vi "Test read mag.vi"() -> ()   [LabVIEW 2013]
uses:
  <vilib>/ni845x/ni845x.llb/ni845xControl.ctl
panel:
  out "whoami 2":u8 format="%.0x"
  out "whoami":u8 format="%.0x"
  out "dt":u32
  out "Waveform Chart":u8[](graph)
  in  "Stop":bool
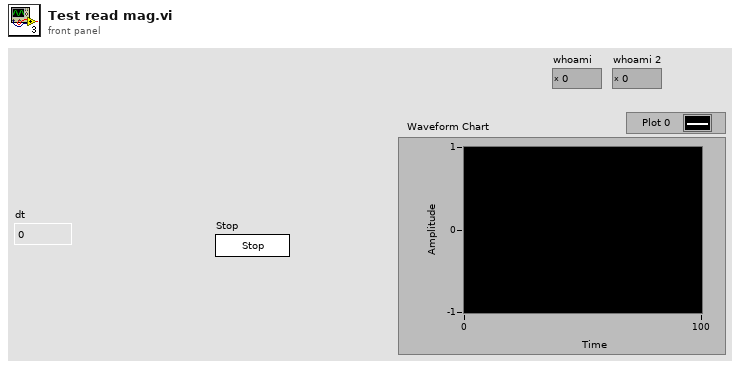
[diagram p1: front panel]
types:
  T1 = typedef "ni845xControl.ctl" = refnum<k21>
  T2 = typedef "AccelerometerSPI.ctl" = cluster{"Device":T1, "spi configuration":T3}
  T3 = typedef "ni845xSpiConfiguration.ctl" = refnum<k20>
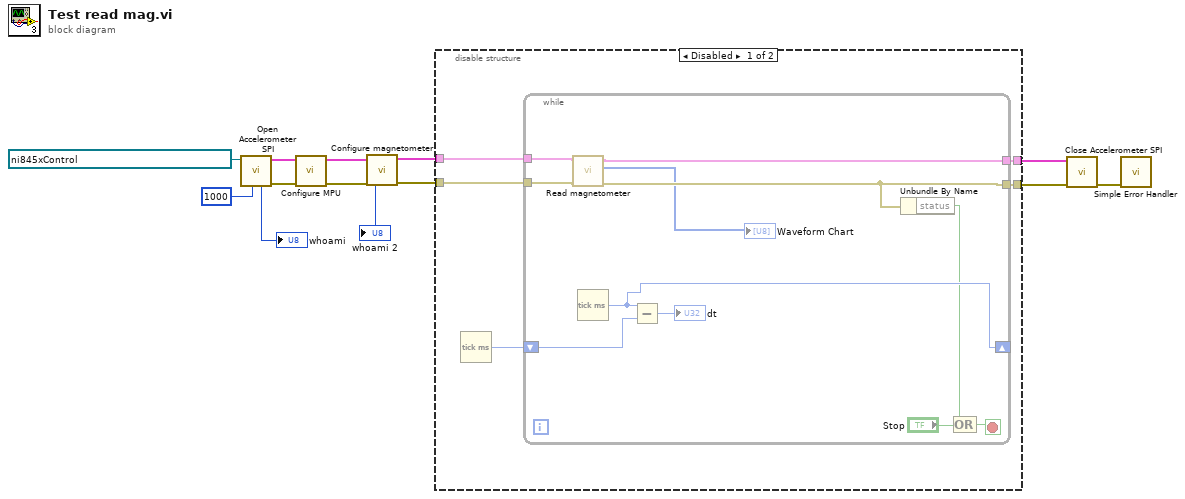
[diagram p0: block diagram]
diagram:
  n1 = call "Open Accelerometer SPI.vi"("Clock Rate in kHz"=u16 1000, "Device"=T1 "USB0::0x3923::0x7166::01879089::RAW") -> ("error out"=w6:errorcluster, "Accelerometer"=w5:T2, "whoami"=→"whoami":u8)  [unwired: 7 in]
  n2 = call "Configure MPU.vi"("error in (no error)"=w6, "Accelerometer"=w5) -> ("error out"=w3:errorcluster, "Accelerometer out"=w4:T2)  [unwired: 8 in]
  n3 = call "Configure magnetometer.vi"("error in (no error)"=w3, "Accelerometer"=w4) -> ("error out"=w1:errorcluster, "Accelerometer out"=w2:T2, "whoami"=→"whoami 2":u8)  [unwired: 7 in]
  n4 = disable-structure shown="Disabled" {
    disable-tunnel: [w18 w31] -> w10
    disable-tunnel: [w17 w30] -> w9
    disable-tunnel: w2 -> [w15 w31]
    disable-tunnel: w1 -> [w14 w30]
    frame Disabled {
      n5 = Tick Count (ms)() -> (millisecond timer value=w16:u32)
      n6 = while {
        tunnel: [w21] -> w18
        tunnel: [w20] -> w17
        tunnel: w15 -> [w23]
        tunnel: w14 -> [w22]
        shift-right: [w28] -> _
        shift-left: w16 -> [w29]
        stop <- w24 stop-if-true
        n7 = call "Read magnetometer.vi"("error in (no error)"=w22, "Accelerometer"=w23) -> ("error out"=w20:errorcluster, "read data"=→"Waveform Chart":u8[], "Accelerometer out"=w21:T2)  [unwired: 7 in]
        n8 = Tick Count (ms)() -> (millisecond timer value=w28:u32)
        n9 = Subtract(x=w28, y=w29) -> (x-y=→"dt":u32)
        n10 = Unbundle By Name(w20) -> ("status"=w25:bool)
        n11 = Compound Arithmetic op=OR(w25, "Stop") -> (w24:bool)
      }
    }
    frame Enabled {
    }
  }
  n12 = call "Close Accelerometer SPI.vi"("error in (no error)"=w9, "Accelerometer"=w10) -> ("error out"=w11:errorcluster)  [unwired: 9 in]
  n13 = call <vilib>:"Simple Error Handler.vi"("error in (no error)"=w11) -> ()  [unwired: 4 in, 5 out]
